vi "GPSCoordCollector.vi"() -> ()   [LabVIEW 2024]
uses:
  <vilib>/Instr/_visa.llb/VISA Configure Serial Port (Instr).vi
panel:
  out "Altitude(m)":dbl
  out "Logitude(deg)":dbl
  out "Latitude(deg)":dbl
  in  "COM7":refnum<visa-resource-name>="COM3" caption="GPS_Com."
  out "True_Heading":dbl format="%#_15g"
  out "UTM X(E) INS":dbl format="%#_13g"
  out "UTM Y(N) INS":dbl format="%#_13g"
  out "GPS_Speed(kph)":dbl format="%#_g kph"
  in  "Stop":bool
  out "NMEA_Raw_Data":string
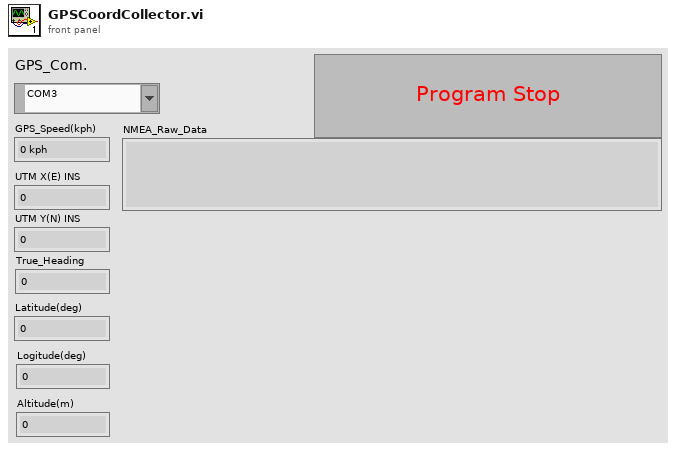
[diagram p1: front panel]
types:
  T1 = cluster{"oldest read timestamp":dbl, "latitude (deg)":dbl, "longitude (deg)":dbl, "ground speed (kph)":dbl, "true track angle (deg)":dbl, "altitude above mean sea level (m)":dbl}
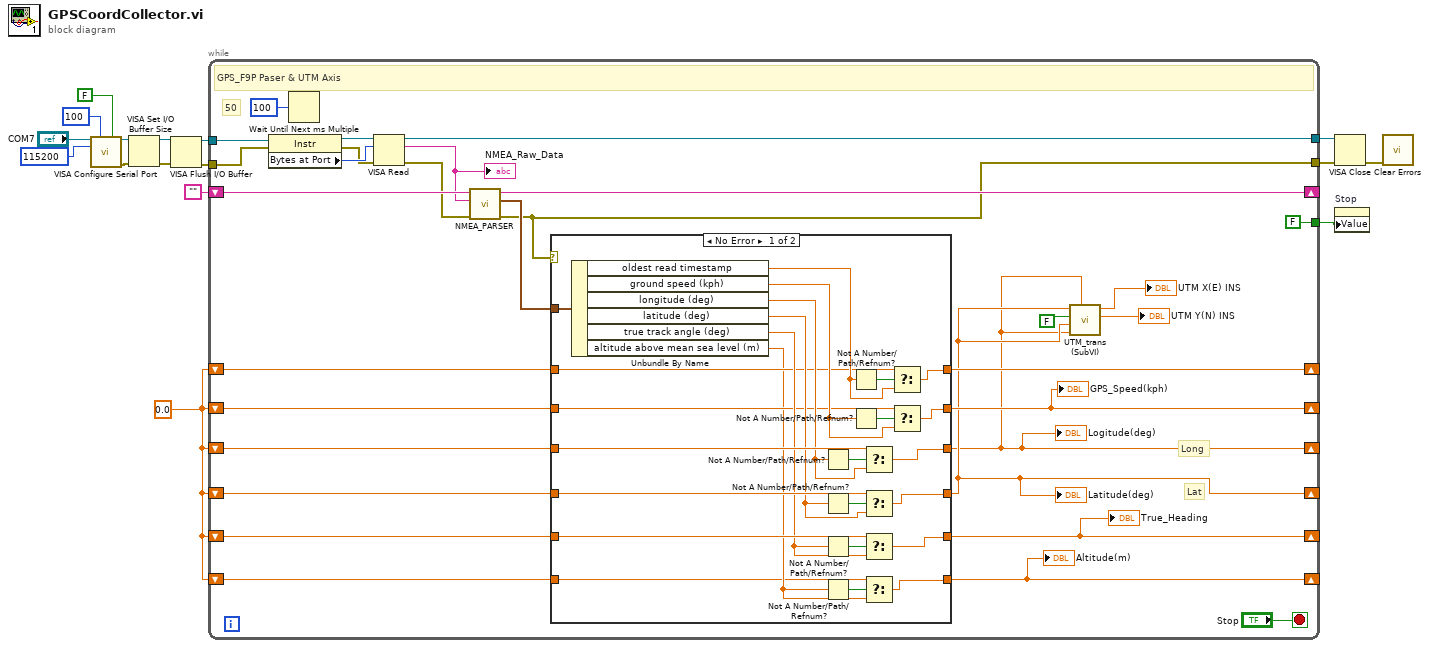
[diagram p0: block diagram]
diagram:
  w1 = 0.0 ("x")
  n1 = call-poly "VISA Configure Serial Port"("VISA resource name"="COM7", "timeout (10sec)"=u32 100, "Enable Termination\nChar (T)"=FALSE ("Enable Termination\nChar (T)"), "baud rate (9600)"=u32 115200) -> ("VISA resource name out"=w7:refnum<visa-resource-name>, "error out"=w6:errorcluster)  [unwired: 10 in]
  n2 = VISA Set I/O Buffer Size(VISA resource name=w7, error in (no error)=w6) -> (VISA resource name out=w13:refnum<visa-resource-name>, error out=w12:errorcluster)  [unwired: 2 in]
  n3 = VISA Flush I/O Buffer(VISA resource name=w13, error in (no error)=w12) -> (VISA resource name out=w11:refnum<visa-resource-name>, error out=w10:errorcluster)  [unwired: 1 in]
  n4 = while {
    tunnel: w11 -> [w44]
    tunnel: w10 -> [w42]
    tunnel: [w46] -> w16
    tunnel: [w34] -> w14
    shift-right: [w35] -> _
    shift-left: "" -> [w39]
    shift-right: [w21] -> _
    shift-left: w1 -> [w33]
    shift-right: [w19] -> _
    shift-left: w1 -> [w32]
    shift-right: [w20] -> _
    shift-left: w1 -> [w31]
    shift-right: [w27] -> _
    shift-left: w1 -> [w30]
    shift-right: [w26] -> _
    shift-left: w1 -> [w29]
    tunnel: [FALSE] -> w8
    shift-right: [w17] -> _
    shift-left: w1 -> [w18]
    stop <- "Stop" stop-if-true
    # "Lat"
    # "Long"
    # "50"
    # "GPS_F9P Paser & UTM Axis"
    n5 = property class="Instr"(reference=w44, error in=w42) -> (reference out=w43:refnum<visa-resource-name>, error out=w41:errorcluster, "Bytes at Port"=w45:u32)
    n6 = Wait Until Next ms Multiple(millisecond multiple=u32 100) -> ()  [unwired: 1 out]
    n7 = VISA Read(VISA resource name=w43, byte count=w45, error in (no error)=w41) -> (VISA resource name out=w46:refnum<visa-resource-name>, read buffer=w38:string, error out=w36:errorcluster)  [unwired: 1 out]
    "NMEA_Raw_Data" <- w38
    n8 = call "NMEA_PARSER.vi"("previous partial sentence"=w39, "sensor data"=w38, "error in (no error)"=w36) -> ("remaining partial sentence"=w35:string, "GPS data"=w37:T1, "error out"=w34:errorcluster)  [unwired: 5 in]
    n9 = case shown="No Error" w34 {
      tunnel: w37 -> [w71 _]
      tunnel: w32 -> [w67 w77]
      tunnel: w31 -> [w66 w76]
      tunnel: w30 -> [w65 w75]
      tunnel: [w61 w77] -> w19
      tunnel: [w60 w76] -> w20
      tunnel: [w59 w75] -> w27
      tunnel: w33 -> [w56 w74]
      tunnel: [w55 w74] -> w21
      tunnel: w29 -> [w52 w73]
      tunnel: [w51 w73] -> w26
      tunnel: [w48 w72] -> w17
      tunnel: w18 -> [w47 w72]
      frame No Error {
        n10 = Unbundle By Name(w71) -> ("oldest read timestamp"=w53:dbl, "ground speed (kph)"=w57:dbl, "longitude (deg)"=w64:dbl, "latitude (deg)"=w63:dbl, "true track angle (deg)"=w62:dbl, "altitude above mean sea level (m)"=w49:dbl)
        n11 = Not A Number/Path/Refnum?(number/path/refnum=w64) -> (NaN/Path/Refnum?=w70:bool)
        n12 = Not A Number/Path/Refnum?(number/path/refnum=w63) -> (NaN/Path/Refnum?=w69:bool)
        n13 = Not A Number/Path/Refnum?(number/path/refnum=w62) -> (NaN/Path/Refnum?=w68:bool)
        n14 = Not A Number/Path/Refnum?(number/path/refnum=w49) -> (NaN/Path/Refnum?=w50:bool)
        n15 = Not A Number/Path/Refnum?(number/path/refnum=w53) -> (NaN/Path/Refnum?=w54:bool)
        n16 = Not A Number/Path/Refnum?(number/path/refnum=w57) -> (NaN/Path/Refnum?=w58:bool)
        n17 = Select(t=w67, s=w70, f=w64) -> (s? t:f=w61:dbl)
        n18 = Select(t=w66, s=w69, f=w63) -> (s? t:f=w60:dbl)
        n19 = Select(t=w65, s=w68, f=w62) -> (s? t:f=w59:dbl)
        n20 = Select(t=w47, s=w50, f=w49) -> (s? t:f=w48:dbl)
        n21 = Select(t=w52, s=w54, f=w53) -> (s? t:f=w51:dbl)
        n22 = Select(t=w56, s=w58, f=w57) -> (s? t:f=w55:dbl)
      }
      frame Error {
        # "Invalid data points."
      }
    }
    "True_Heading" <- w27
    "GPS_Speed(kph)" <- w21
    "Latitude(deg)" <- w20
    "Logitude(deg)" <- w19
    "Altitude(m)" <- w17
    n23 = call "UTM_trans (SubVI).vi"("Long_Deg"=w19, "long"=w19, "lat"=w20, "East?West?"=FALSE, "Lat_Deg"=w20) -> ("UTM_Y(Northing)"=→"UTM Y(N) INS":dbl, "UTM_X(Easting)"=→"UTM X(E) INS":dbl)  [unwired: 2 out]
  }
  n24 = VISA Close(VISA resource name=w16, error in (no error)=w14) -> (error out=w15:errorcluster)
  n25 = property on="Stop" class="Bool (strict)"("Value"=w8) -> ()  [unwired: 2 in, 2 out]
  n26 = call <vilib>:"Clear Errors.vi"("error in (no error)"=w15) -> ()  [unwired: 5 in, 2 out]
